vi "Get Filtered Components.vi"(5 "Device Class":string, 6 "Product ID":i32 format="%.0x", 7 "Operating System":string, 8 "error in (no error)":errorcluster, 10 "Item Types (all visible)":T3 items=["all visible", "all including hidden", "standard only", "startup only"], 11 "Repository in (RT Images)":path) -> (0 "error out":errorcluster, 2 "Software Components":T1[](array[typedef]) {"component type" items=["standard", "hidden", "system", "unknown", "startup", "image"]}, 3 "Repository out":path)   [LabVIEW 2012, in "nisyscfg.lvlib"]
doc: "Retrieves a list of software components on the local system that are available for installation to the specified target."
uses:
  <vilib>/nisyscfg/nisyscfg.lvlib
  <vilib>/nisyscfg/Component Types.ctl
  <vilib>/nisyscfg/Software 1.2.ctl
  <vilib>/nisyscfg/Component Type.ctl
  <resource>/objmgr/nisysapi.rc
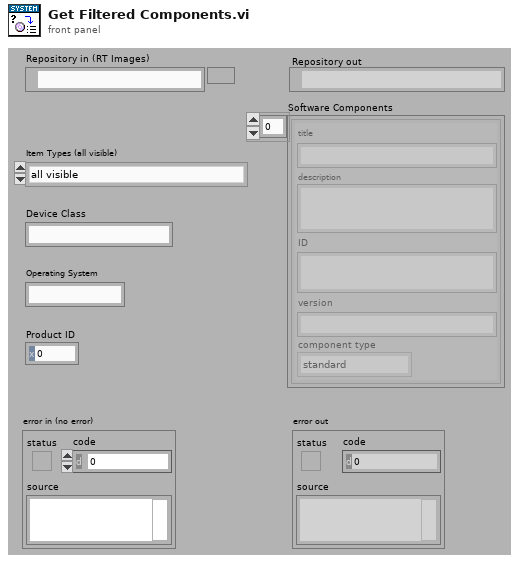
[diagram p1: front panel]
types:
  T1 = typedef "nisyscfg.lvlib/Software 1.2.ctl" = cluster{"title":string, "description":string, "ID":string, "version":string, "component type":T2}
  T2 = typedef "nisyscfg.lvlib/Component Type.ctl" = u32
  T3 = typedef "nisyscfg.lvlib/Component Types.ctl" = u32
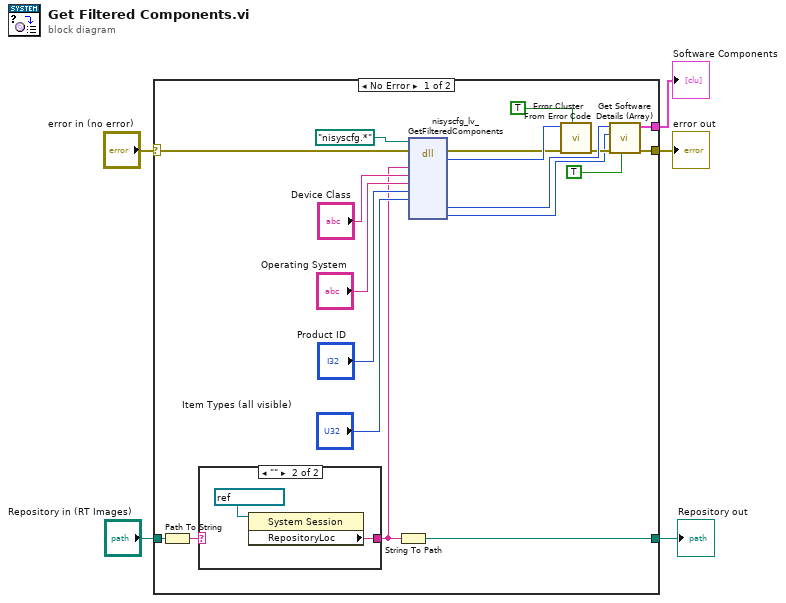
[diagram p0: block diagram]
diagram:
  n1 = case shown="No Error" "error in (no error)" {
    selector: "error in (no error)" -> [w22 w29]
    tunnel: [w17 w29] -> w5
    tunnel: "Repository in (RT Images)" -> [w9 w28]
    tunnel: [w16 _] -> w2
    tunnel: [w6 w28] -> w1
    frame No Error {
      n2 = Path To String(path=w9) -> (string=w8:string)
      n3 = case shown="\"\"" w8 {
        selector: w8 -> [w25 _]
        tunnel: [w25 w27] -> w7
        frame Default {
        }
        frame "" {
          n4 = property class="System Session"(reference=refnum<k21> "localhost" ("System Configuration")) -> ("RepositoryLoc"=w27:string)  [unwired: 1 in, 2 out]
        }
      }
      n5 = String To Path(string=w7) -> (path=w6:path)
      n6 = dll-call lib="nisyscfg.*" fn="nisyscfg_lv_GetFilteredComponents" label="GetFilteredComponents"(path in=path "nisyscfg.*", error in=w22, "repository"=w7, "deviceClass"="Device Class", "operatingSystem"="Operating System", "productID"="Product ID", "itemTypes"="Item Types (all visible)") -> (error out=w23:errorcluster, "result"=w24:i32, "components"=w19:u64, "numComponents"=w15:i32)  [unwired: 8 in, 1 out]
      n7 = call <vilib>:"Error Cluster From Error Code.vi"("show call chain? (False)"=TRUE, "error in (no error)"=w23, "error code (0)"=w24) -> ("error out"=w18:errorcluster)  [unwired: 6 in]
      n8 = call <vilib>:"Get Software Details (Array).vi"("Trace Component Info (F)"=TRUE ("log to NI Spy (F)"), "error in (no error)"=w18, "Number of Elements"=w15, "Enumerator in"=w19) -> ("error out"=w17:errorcluster, "Software Components"=w16:T1[])  [unwired: 6 in]
    }
    frame Error {
    }
  }
  "error out" <- w5
  "Software Components" <- w2
  "Repository out" <- w1
